vi "Read.vi"(6 "Append Index":i32, 8 "error in (no error)":errorcluster, 11 "Data.S3":refnum<class "Data.S3.lvclass">) -> (0 "error out":errorcluster, 1 "Notes":string, 2 "Data (Dictionary)":T1[](array[typedef]), 3 "Data.S3 out":refnum<class "Data.S3.lvclass">, 5 "Path out":path)   [LabVIEW 2016, in "Data.S3.lvclass"]
uses:
  Data.S3.lvclass
  Data/Typedefs/Dictionary--cluster.ctl
  Data/Data.lvclass
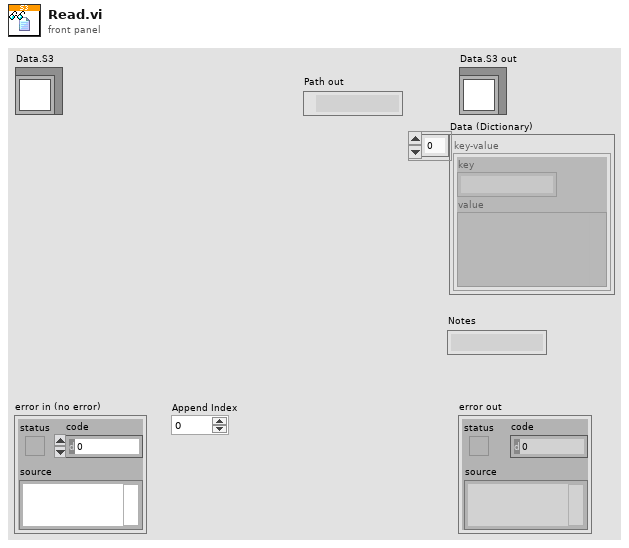
[diagram p1: front panel]
types:
  T1 = typedef "Data.lvclass/Dictionary--cluster.ctl" = cluster{"key":string, "value":variant}
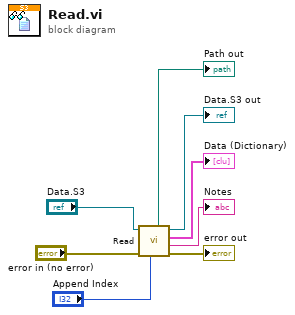
[diagram p0: block diagram]
diagram:
  n1 = call-parent "Read.vi"("Append Index"="Append Index", "error in (no error)"="error in (no error)", "Data Save in"="Data.S3") -> ("error out"=→"error out":errorcluster, "Notes"=→"Notes":string, "Data (Dictionary)"=→"Data (Dictionary)":T1[], "Data Save out"=→"Data.S3 out":refnum<class "Data.S3.lvclass">, "Path out"=→"Path out":path)  [unwired: 4 in]
